vi "SetSignalParams.vi"(8 "error in (no error)":errorcluster, 10 "Variant":variant, 11 "StandardFunction in":refnum<class "StandardFunction.lvclass">) -> (0 "error out":errorcluster, 3 "StandardFunction out":refnum<class "StandardFunction.lvclass">)   [LabVIEW 2018, in "Functions.lvlib" / "StandardFunction.lvclass"]
uses:
  StandardFunction.lvclass
  StandardFunction.lvclass/StandardFunction.ctl
  TypeDefs/StdWfrm.ctl
  Accessors/Read StandardWfrms.vi
  Accessors/Write StandardWfrms.vi
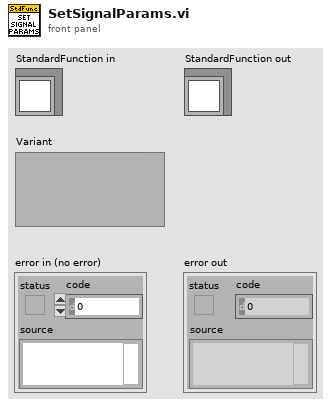
[diagram p1: front panel]
types:
  T1 = typedef "Functions.lvlib/StandardFunction.lvclass/StdWfrm.ctl" = cluster{"Amplitude":dbl, "DcOffset":dbl, "DutyCycle":dbl, "Frequency":dbl, "Phase":dbl, "Waveform":enum16{"Sine", "Square", "Triangle", "Ramp Up", "Ramp Down", "DC"}, "Handle":string}
  T2 = typedef "Functions.lvlib/StandardFunction.lvclass/StdWfrms.ctl" = cluster{"Count":u16, "StandardWfrm":T1[]}
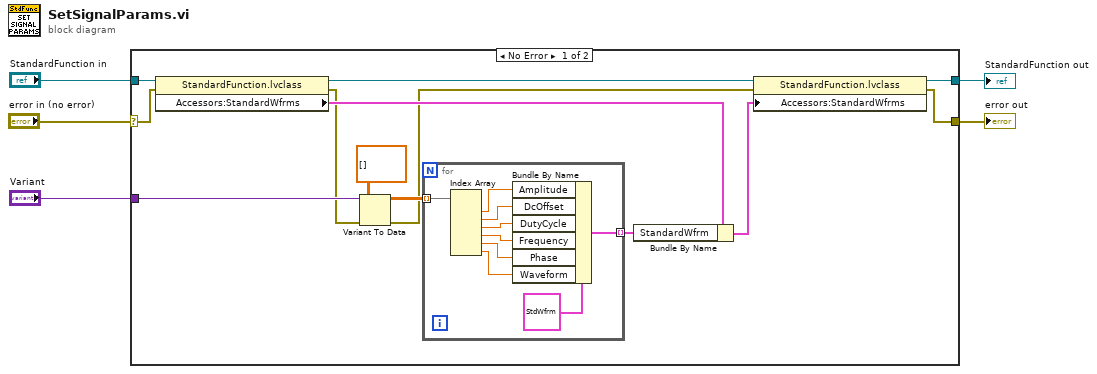
[diagram p0: block diagram]
diagram:
  n1 = case shown="No Error" "error in (no error)" {
    selector: "error in (no error)" -> [w14 w28]
    tunnel: "StandardFunction in" -> [w15 w29]
    tunnel: [w7 w29] -> w3
    tunnel: [w6 w28] -> w2
    tunnel: "Variant" -> [w18 _]
    frame No Error {
      n2 = property class="StandardFunction.lvclass"(reference=w15, error in=w14) -> (reference out=w10:refnum<class "StandardFunction.lvclass">, error out=w11:errorcluster, "Accessors:StandardWfrms"=w13:T2)
      n3 = Variant To Data(error in=w11, type=dbl[][] [], Variant=w18) -> (data=w16:dbl[][], error out=w8:errorcluster)
      n4 = for {
        tunnel: w16 -> [w26] mode=indexing
        tunnel: [w19] -> w12 mode=indexing
        n5 = Index Array(array=w26) -> (element #1=w25:dbl, element #2=w24:dbl, element #3=w23:dbl, element #4=w22:dbl, element #5=w20:dbl, element #6=w21:dbl)  [unwired: 6 in]
        n6 = Bundle By Name(cluster=T1 {"Amplitude"=0.0, "DcOffset"=0.0, "DutyCycle"=0.0, "Frequency"=0.0, "Phase"=0.0, "Waveform"=enum."Sine", "Handle"=""} ("StandardWfrm"), "Amplitude"=w25, "DcOffset"=w24, "DutyCycle"=w23, "Frequency"=w22, "Phase"=w20, "Waveform"=w21) -> (w19:T1)
      }
      n7 = Bundle By Name(cluster=w13, "StandardWfrm"=w12) -> (w9:T2)
      n8 = property class="StandardFunction.lvclass"(reference=w10, error in=w8, "Accessors:StandardWfrms"=w9) -> (reference out=w7:refnum<class "StandardFunction.lvclass">, error out=w6:errorcluster)
    }
    frame Error {
    }
  }
  "error out" <- w2
  "StandardFunction out" <- w3
